vi "Delete.vi"   [LabVIEW 2020, in "OXYGEN_Datastream.lvlib"]
uses:
  OXYGEN_Datastream.lvlib
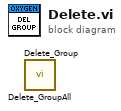
[diagram p0: block diagram]
diagram:
  n1 = call "Delete_GroupAll.vi"() -> ()  [unwired: 9 in, 3 out]
  n2 = call "Delete_Group.vi"() -> ()  [unwired: 9 in, 3 out]
